vi "Set Manual.vi"(10 "Manual":bool, 11 "PIDClass.lvclass":refnum<class "PIDClass.lvclass">) -> (3 "PIDClass.lvclass out":refnum<class "PIDClass.lvclass">)   [LabVIEW 2012, in "PIDClass.lvclass"]
uses:
  PIDClass.lvclass
  PIDClass.lvclass/PIDClass.ctl
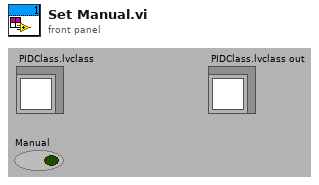
[diagram p1: front panel]
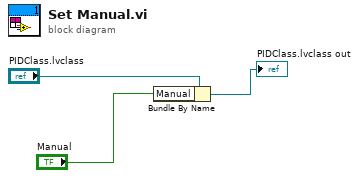
[diagram p0: block diagram]
diagram:
  n1 = Bundle By Name(cluster="PIDClass.lvclass", "Manual"="Manual") -> (→"PIDClass.lvclass out":refnum<class "PIDClass.lvclass">)
